vi "v6.1.vi"() -> ()   [LabVIEW 2018]
uses:
  <vilib>/DAQmx/read.llb/DAQmx Read (Analog 1D DBL NChan 1Samp).vi
  <extravilib>/ChannelInstances/Lossy Stream-c(a[.](c(dbl,dbl,dbl,dbl)),stamp,a[.](dbl),c(dbl,dbl,dbl,dbl,dbl,dbl,dbl))/Read With Abort.vi
  <extravilib>/ChannelInstances/High Speed Stream-c(a[.](c(dbl,dbl,dbl,dbl)),stamp,a[.](dbl),c(dbl,dbl,dbl,dbl,dbl,dbl,dbl))/_Read For Replicate.vi
  <extravilib>/ChannelInstances/Lossy Stream-c(a[.](c(dbl,dbl,dbl,dbl)),stamp,a[.](dbl),c(dbl,dbl,dbl,dbl,dbl,dbl,dbl))/Write With Abort.vi
  <extravilib>/ChannelInstances/Lossy Stream-c(a[.](c(dbl,dbl,dbl,dbl)),stamp,a[.](dbl),c(dbl,dbl,dbl,dbl,dbl,dbl,dbl))/EndpointRead.vi
  <extravilib>/ChannelInstances/Lossy Stream-c(a[.](c(dbl,dbl,dbl,dbl)),stamp,a[.](dbl),c(dbl,dbl,dbl,dbl,dbl,dbl,dbl))/Endpoint.vi
  <extravilib>/ChannelInstances/Lossy Stream-c(a[.](c(dbl,dbl,dbl,dbl)),stamp,a[.](dbl),c(dbl,dbl,dbl,dbl,dbl,dbl,dbl))/Instantiate.vi
  <extravilib>/ChannelInstances/Lossy Stream-c(a[.](c(dbl,dbl,dbl,dbl)),stamp,a[.](dbl),c(dbl,dbl,dbl,dbl,dbl,dbl,dbl))/)Channel.vi
  <resource>/ChannelSupport/_ChannelSupport/WaitIfNeeded.vi
  <extravilib>/ChannelInstances/High Speed Stream-c(a[.](c(dbl,dbl,dbl,dbl)),stamp,a[.](dbl),c(dbl,dbl,dbl,dbl,dbl,dbl,dbl))/Instantiate.vi
  <extravilib>/ChannelInstances/High Speed Stream-c(a[.](c(dbl,dbl,dbl,dbl)),stamp,a[.](dbl),c(dbl,dbl,dbl,dbl,dbl,dbl,dbl))/)Channel.vi
  <extravilib>/ChannelInstances/High Speed Stream-c(a[.](c(dbl,dbl,dbl,dbl)),stamp,a[.](dbl),c(dbl,dbl,dbl,dbl,dbl,dbl,dbl))/Abort Signal/Init Signal.vi
  <vilib>/Utility/file.llb/Write Delimited Spreadsheet (string).vi
  <vilib>/DAQmx/create/channels.llb/DAQmx Create Channel (AI-Temperature-Thermocouple).vi
  <vilib>/DAQmx/configure/timing.llb/DAQmx Timing (Sample Clock).vi
  <vilib>/DAQmx/miscellaneous.llb/DAQmx Fill In Error Info.vi
  <extravilib>/ChannelInstances/High Speed Stream-c(a[.](c(dbl,dbl,dbl,dbl)),stamp,a[.](dbl),c(dbl,dbl,dbl,dbl,dbl,dbl,dbl)).lvlib
  <resource>/objmgr/daqmx.rc
  <extravilib>/ChannelInstances/Lossy Stream-c(a[.](c(dbl,dbl,dbl,dbl)),stamp,a[.](dbl),c(dbl,dbl,dbl,dbl,dbl,dbl,dbl)).lvlib
panel:
  out "Driving Variables":T1
  in  "Line Controls\n(Don't Delete)":enum32{"Flowrate", "Temperatures", "Pressures"}(tab)
  in  "Line Flowrate Control":T2 {"Line 5" scale=0.0..10.0; "Line 4" scale=0.0..10.0; "Line 3" scale=0.0..10.0; "Line 2" scale=0.0..10.0; "Line 1" scale=0.0..10.0}
  in  "Temperatures Control":T2 {"Line 5" scale=0.0..10.0; "Line 4" scale=0.0..10.0; "Line 3" scale=0.0..10.0; "Line 2" scale=0.0..10.0; "Line 1" scale=0.0..10.0}
  in  "Pressure Controls":T2 {"Line 5" scale=0.0..10.0; "Line 4" scale=0.0..10.0; "Line 3" scale=0.0..10.0; "Line 2" scale=0.0..10.0; "Line 1" scale=0.0..10.0}
  in  "Rig Temperature Tab Box\n(Don't Delete)":enum32{"Rig Temps Live", "Alarm Thresholds"}(tab)
  out "Rig Temperatures":T3
  in  "Rig Alarm Thresholds":T3
  out "DAQ Current Time":timestamp format="%<%X>T"
  in  "UI Refresh Rate (Hz)":u32=1 min=1 max=500 step=1
  out "Line Pressures":T4(graph)
  out "Line Temperatures":T4(graph)
  in  "Species List":string[][](table)=[["Custom", "9999999999", ""], ["Methanol", "6.47", "19.93"], ["Butanol", "11.2", "33.075"], ["Propane", "15.67", "46.35"], ["Methane", "13.19", "50.00"], ["Hydrogen", "34.3", "119.96"], ["Ammonia", "6.0466", "22.5"], ["Pentane", "15.32", "45.36"], ["Butane", "14.98", "45.75"], ["Hexane", "15.24", "44.75"], ["Ethanol", "9", "26.70"], ["Empty (Not Used)", "0", "0"]]
  in  "Lines Tab Control\n(Don't delete)":enum32{"Live Data", "AFR Info", "Setup Lines"}(tab)
  out "Flowrate Data":T5(array[cluster])
  out "AFR Display":T6(array[cluster])
  in  "Line Setup":T7(array[cluster])
  out "Actual Sample Rate":dbl
  out "Export Timestamp":timestamp format="%<%H:%M:%S>T"
  out "UI Timestamp":timestamp format="%<%X\n%x>T"
  in  "file path (dialog if empty)":path
  out "Export Loop Status":T8(ring)
  in  "Start Recording?":bool
  in  "Stop Recording?":bool
  out "Aquisition Loop Status":T9(ring)
  in  "OK Button":bool
  in  "DAQ Properties":cluster{"Sample Rate [Hz]":dbl}={"Sample Rate [Hz]"=1.0} {"Sample Rate [Hz]" min=1.0 max=500.0 step=1.0}
  # "Loop Status"
  # "Rig Temperatures [ °C]"
  # "Rig Alarm Thresholds [ °C]"
  # "Live \n Live Line Data"
  # "Air-to-Fuel Ratios for each Line"
  # "Line Setup"
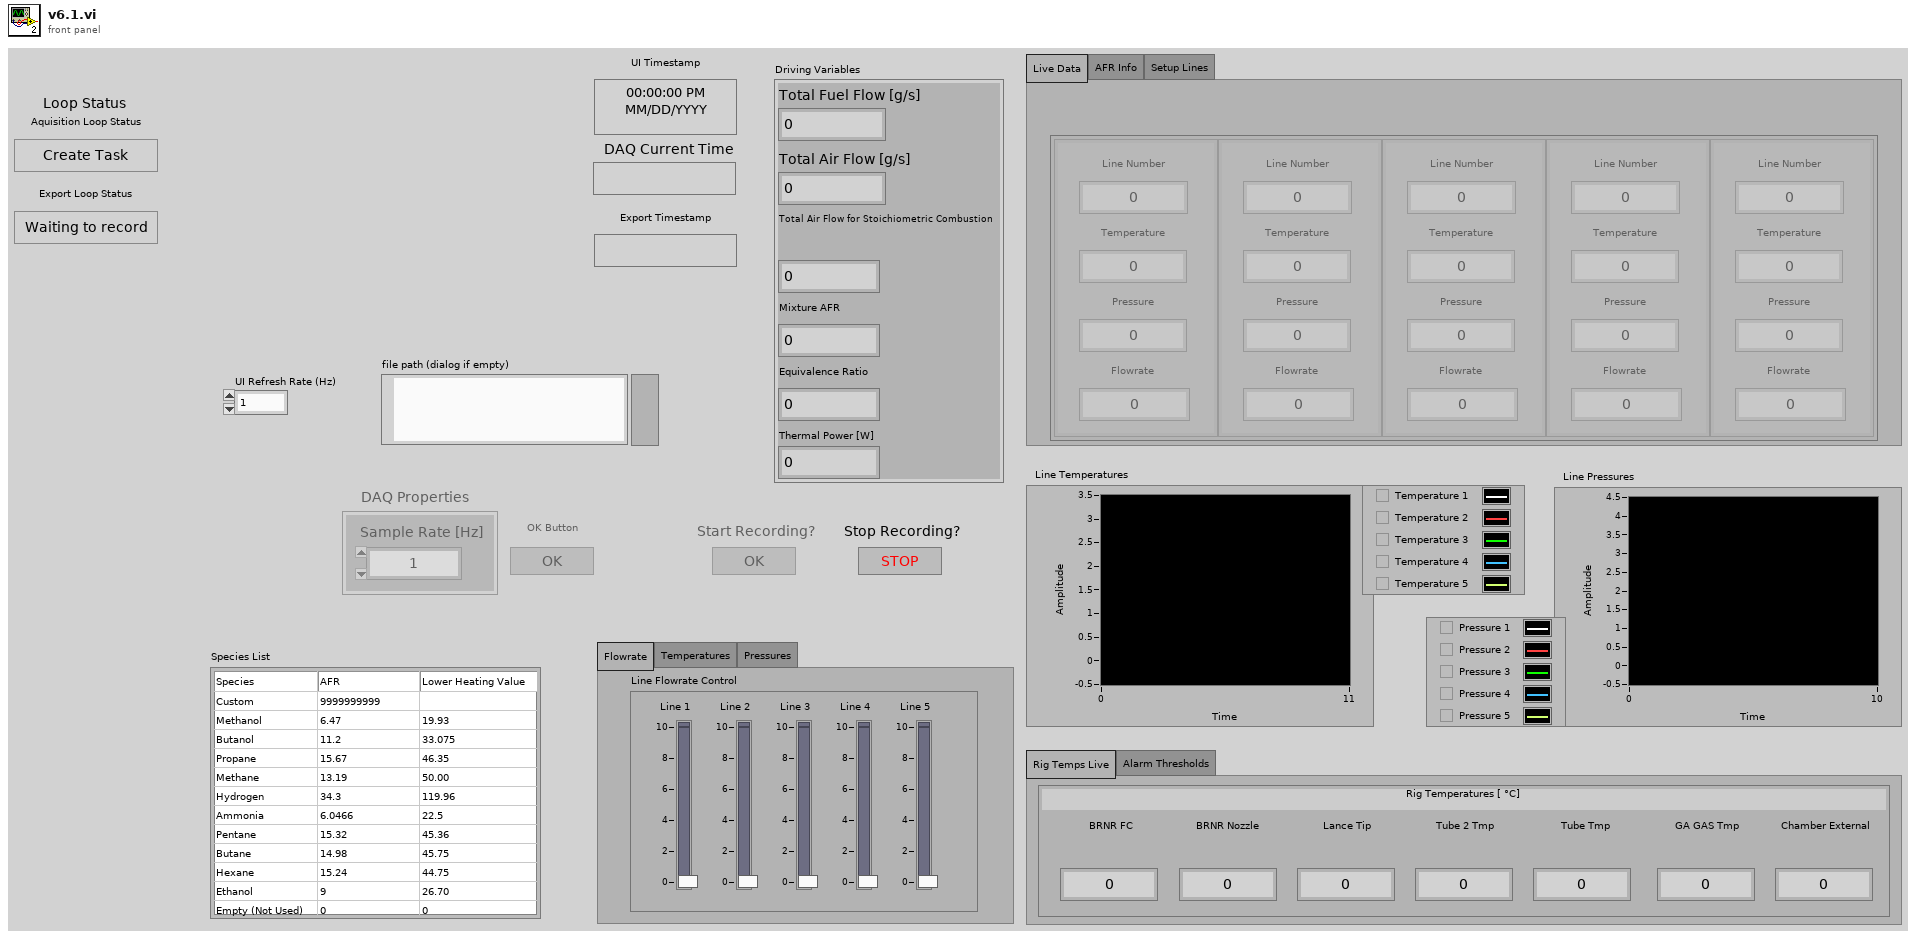
[diagram p1: front panel]
types:
  T1 = cluster{"Total Air Flow [g/s]":dbl, "Total Fuel Flow [g/s]":dbl, "Mixture AFR":dbl, "Total Air Flow for Stoichiometric Combustion":dbl, "Equivalence Ratio":dbl, "Thermal Power [W]":dbl}
  T2 = cluster{"Line 1":dbl, "Line 2":dbl, "Line 3":dbl, "Line 4":dbl, "Line 5":dbl}
  T3 = cluster{"BRNR FC":dbl, "BRNR Nozzle":dbl, "Lance Tip":dbl, "Tube 2 Tmp":dbl, "Tube Tmp":dbl, "GA GAS Tmp":dbl, "Chamber External":dbl}
  T4 = cluster{"[0]":dbl, "[1]":dbl, "[2]":dbl, "[3]":dbl, "[4]":dbl}
  T5 = cluster{"Line Number":dbl, "Temperature":dbl, "Pressure":dbl, "Flowrate":dbl}[]
  T6 = cluster{"Line Number":i32, "AFR":dbl, "Species":enum16{"Empty (Not used)", "Custom", "Air", "Methanol", "Ethanol", "Butanol", "Propane", "Methane", "Hydrogen", "Pentane", "Butane", "Hexane"}}[]
  T7 = cluster{"Custom AFR":dbl, "Species":enum16{"Empty (Not used)", "Custom", "Air", "Methanol", "Ethanol", "Butanol", "Propane", "Methane", "Hydrogen", "Pentane", "Butane", "Hexane"}, "Custom Lower Heating Value [kJ/kg]":dbl}[]
  T8 = enum16{"Waiting to record", "Creating Spreadsheet", "Recording", "Finished Recording"}
  T9 = enum16{"Create Task", "Change Settings", "Check Settings", "Read Data", "End Task"}
  T10 = enum8{"Enabled", "Disabled", "Disabled and Grayed Out"}
  T11 = cluster{"Flowrate Data":cluster{"Line Number":dbl, "Temperature":dbl, "Pressure":dbl, "Flowrate":dbl}[], "Current Time":timestamp, "DAQmx Data":dbl[], "Rig Temperatures":cluster{"BRNR FC":dbl, "BRNR Nozzle":dbl, "Lance Tip":dbl, "Tube 2 Tmp":dbl, "Tube Tmp":dbl, "GA GAS Tmp":dbl, "Chamber External Temp":dbl}}
  T12 = cluster{"BRNR FC":dbl, "BRNR Nozzle":dbl, "Lance Tip":dbl, "Tube 2 Tmp":dbl, "Tube Tmp":dbl, "GA GAS Tmp":dbl, "Chamber External Temp":dbl}
  T13 = typedef "High Speed Stream-c(a[.](c(dbl,dbl,dbl,dbl)),stamp,a[.](dbl),c(dbl,dbl,dbl,dbl,dbl,dbl,dbl)).lvlib/)Channel.ctl" = refnum<queue>
  T14 = typedef "Lossy Stream-c(a[.](c(dbl,dbl,dbl,dbl)),stamp,a[.](dbl),c(dbl,dbl,dbl,dbl,dbl,dbl,dbl)).lvlib/)Channel.ctl" = refnum<queue>
  T15 = cluster{"Line":i32, "AFR":dbl, "Species":enum16{"Empty (Not used)", "Custom", "Air", "Methanol", "Ethanol", "Butanol", "Propane", "Methane", "Hydrogen", "Pentane", "Butane", "Hexane"}}
  T16 = enum16{"Empty (Not used)", "Custom", "Air", "Methanol", "Ethanol", "Butanol", "Propane", "Methane", "Hydrogen", "Pentane", "Butane", "Hexane"}
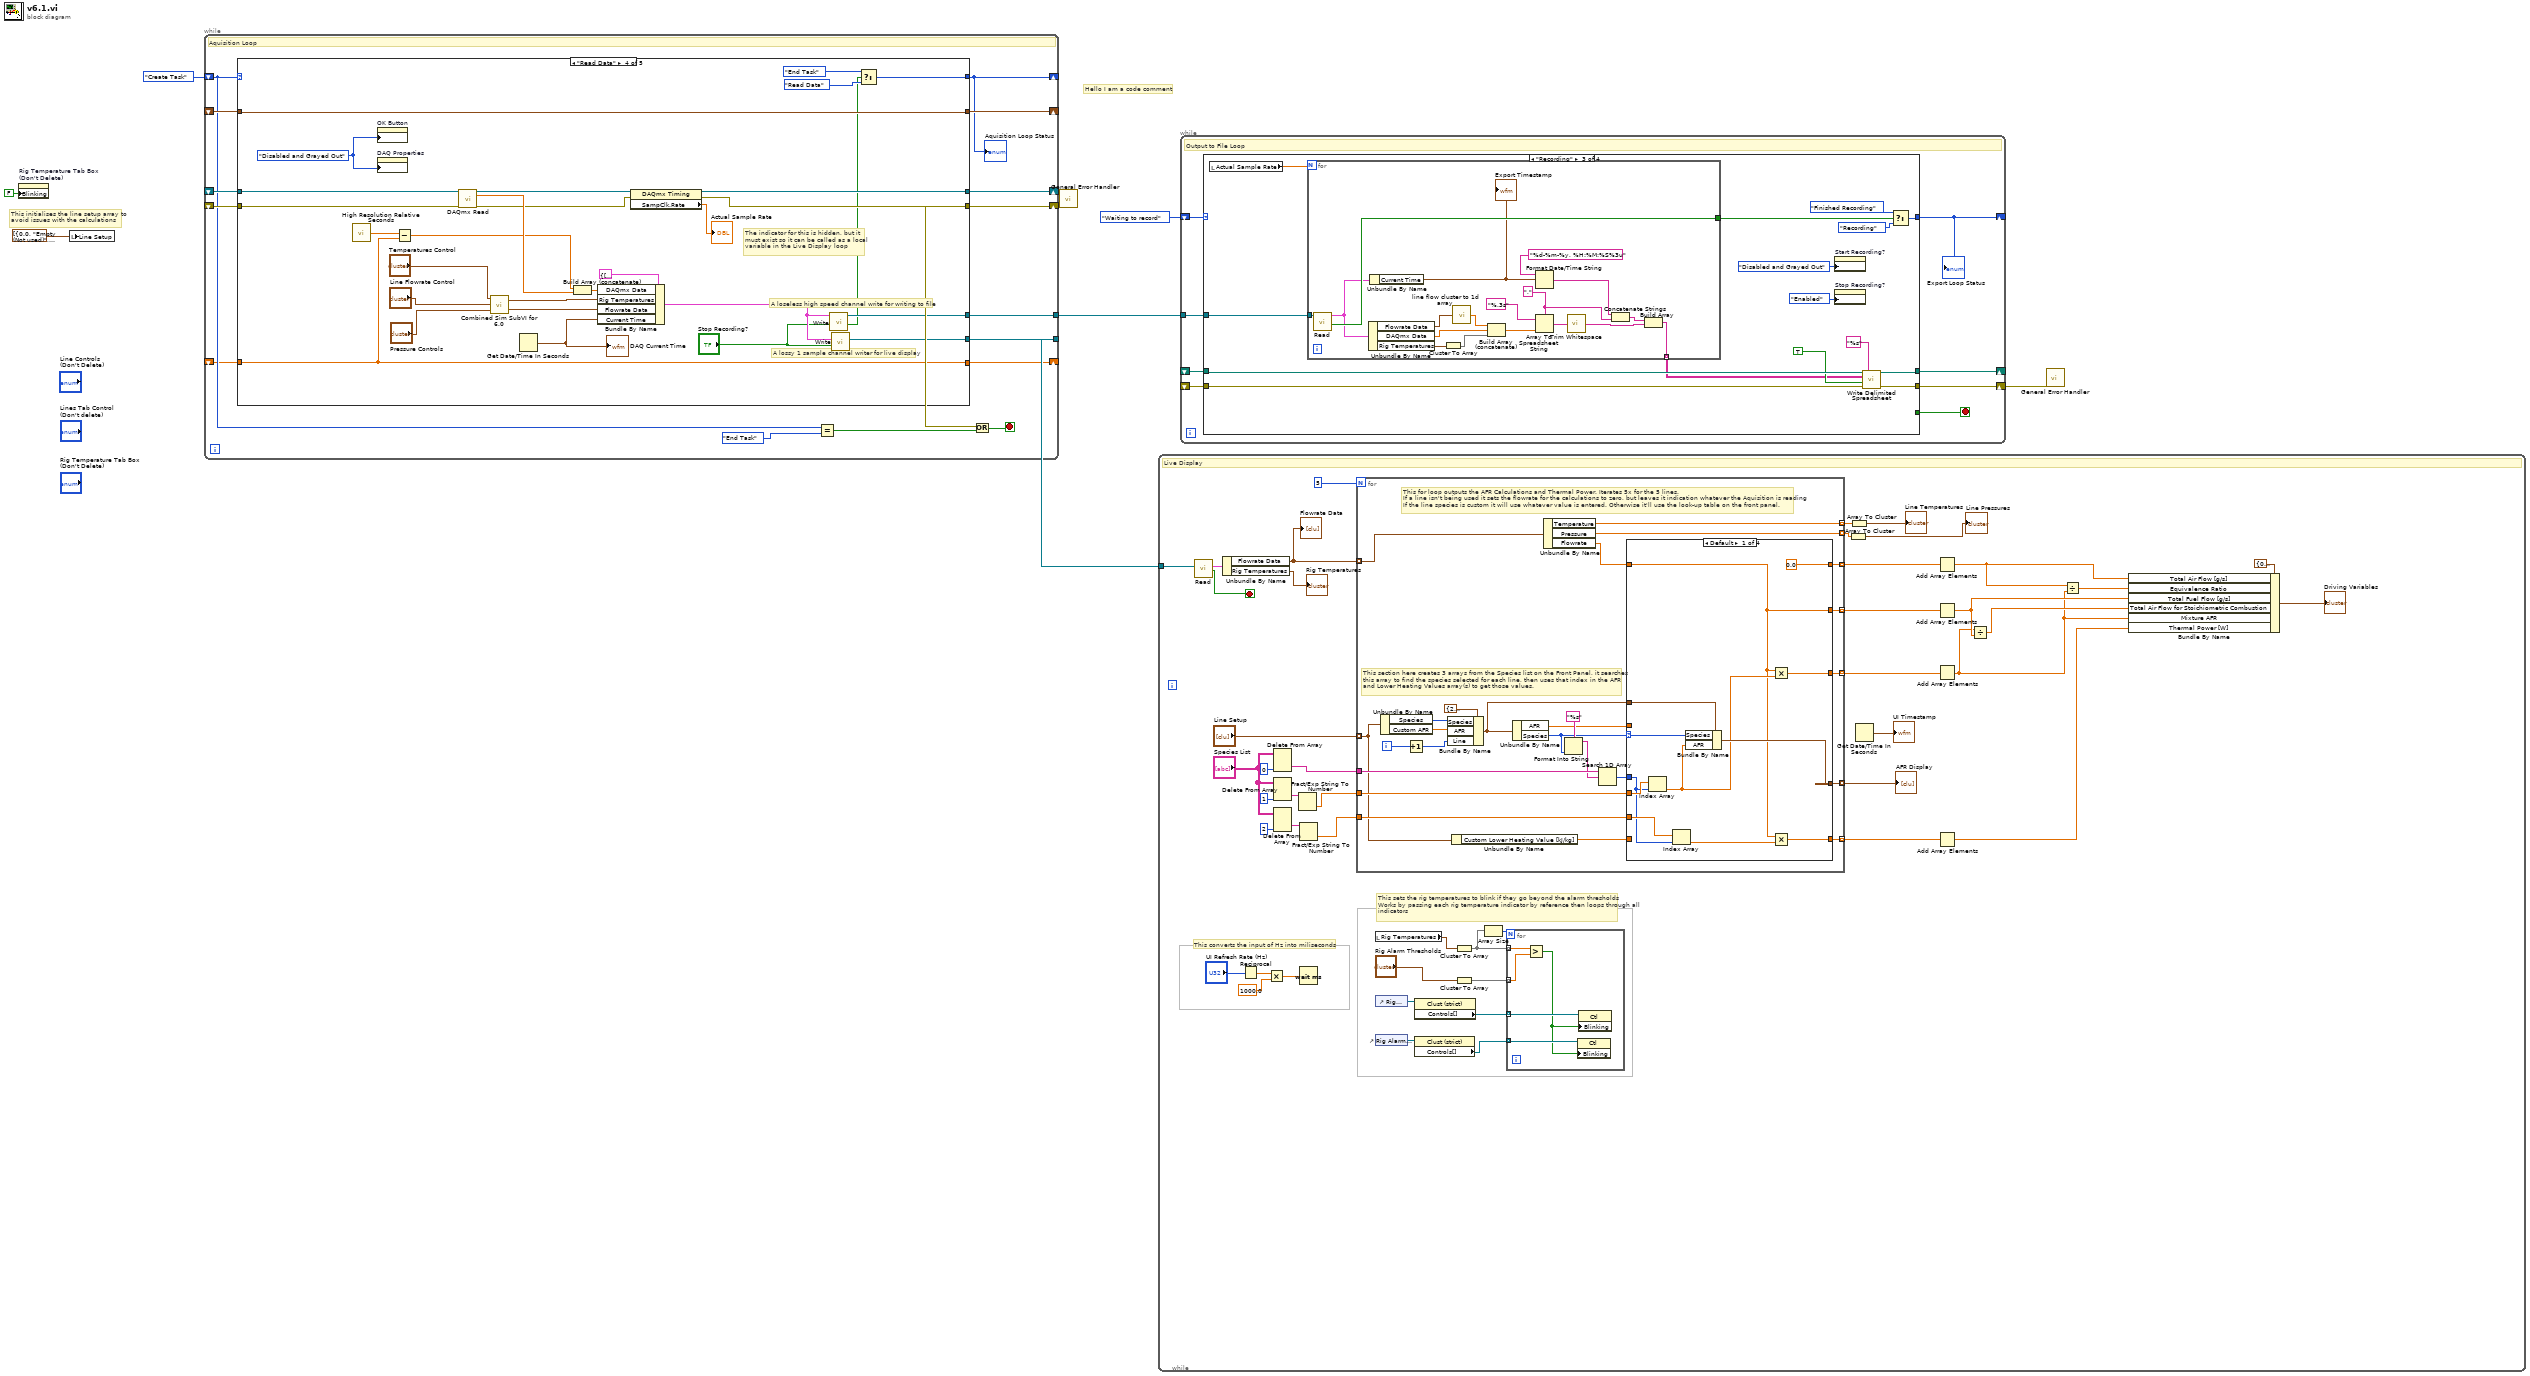
[diagram p0: block diagram]
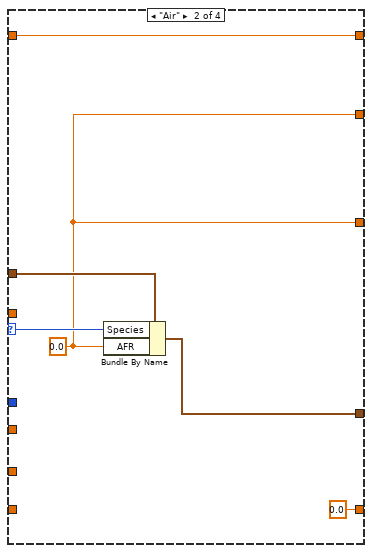
[diagram p2: hidden frame]
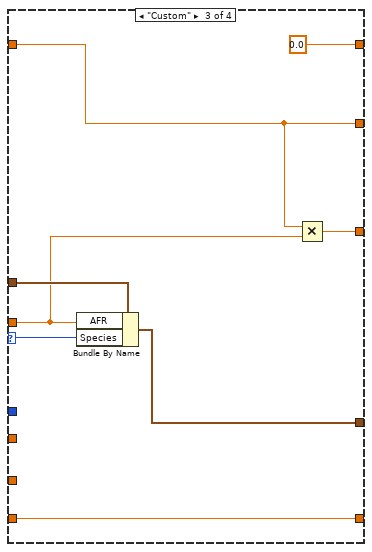
[diagram p3: hidden frame]
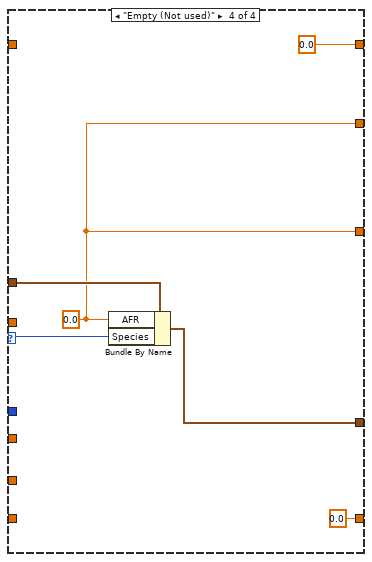
[diagram p4: hidden frame]
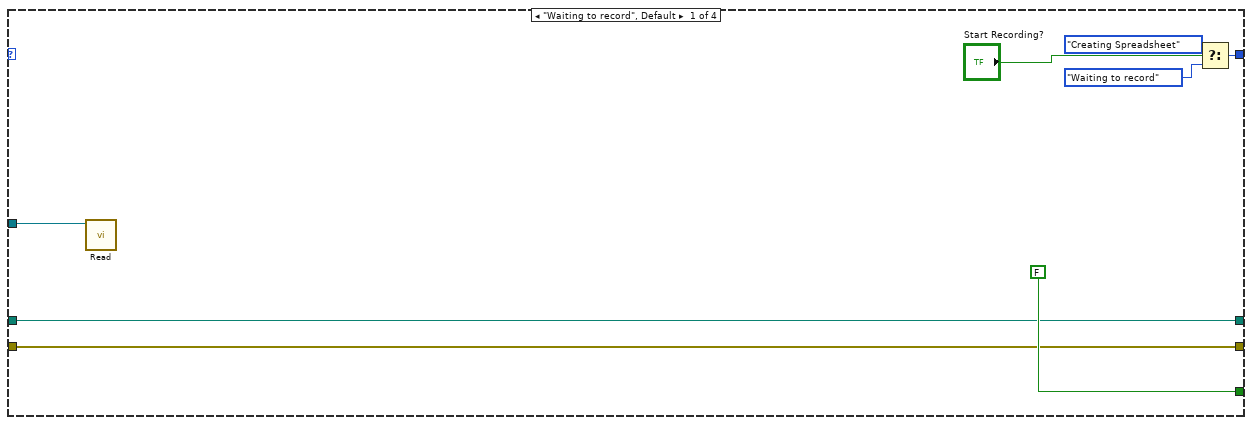
[diagram p5: hidden frame]
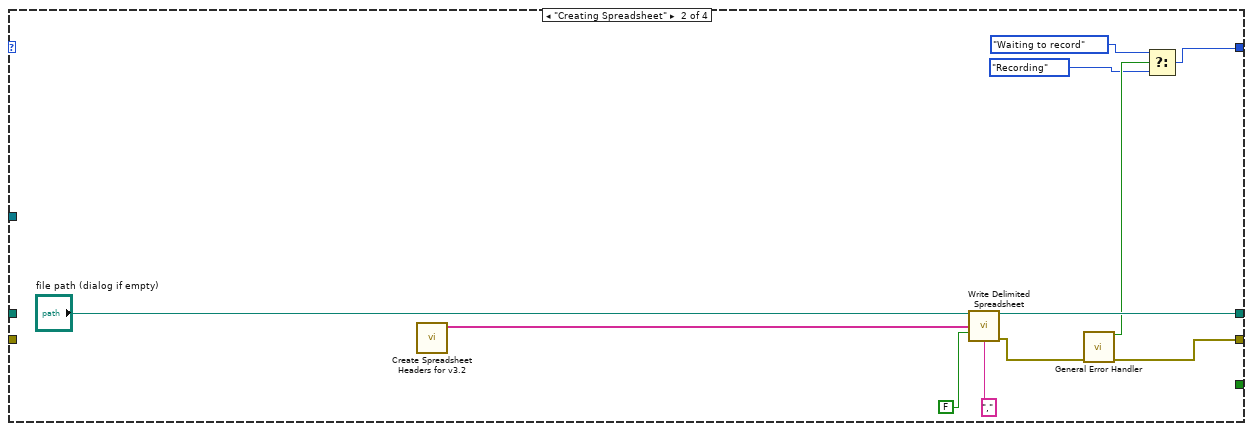
[diagram p6: hidden frame]
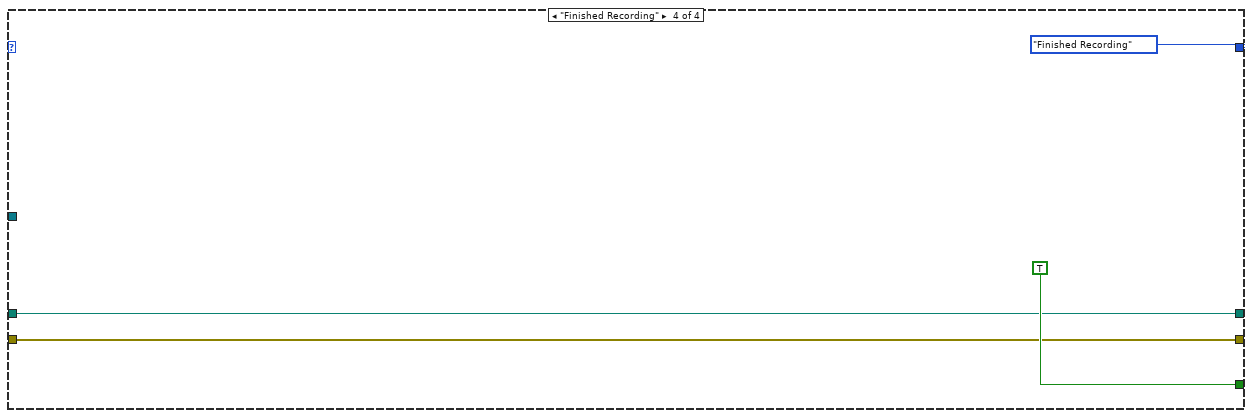
[diagram p7: hidden frame]
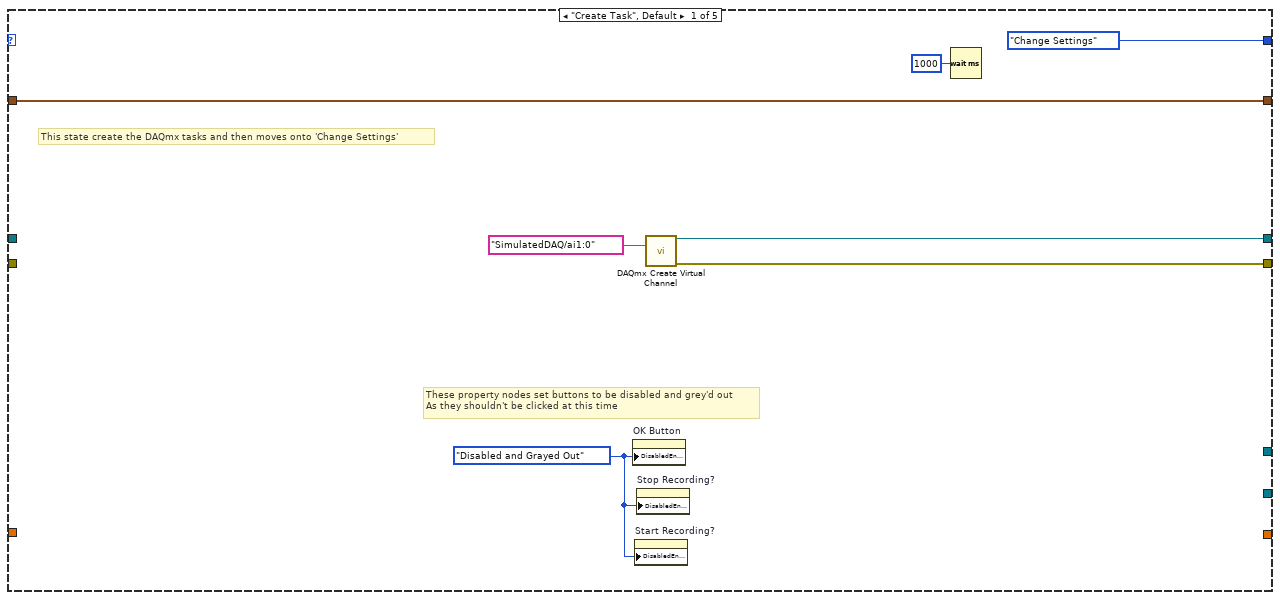
[diagram p8: hidden frame]
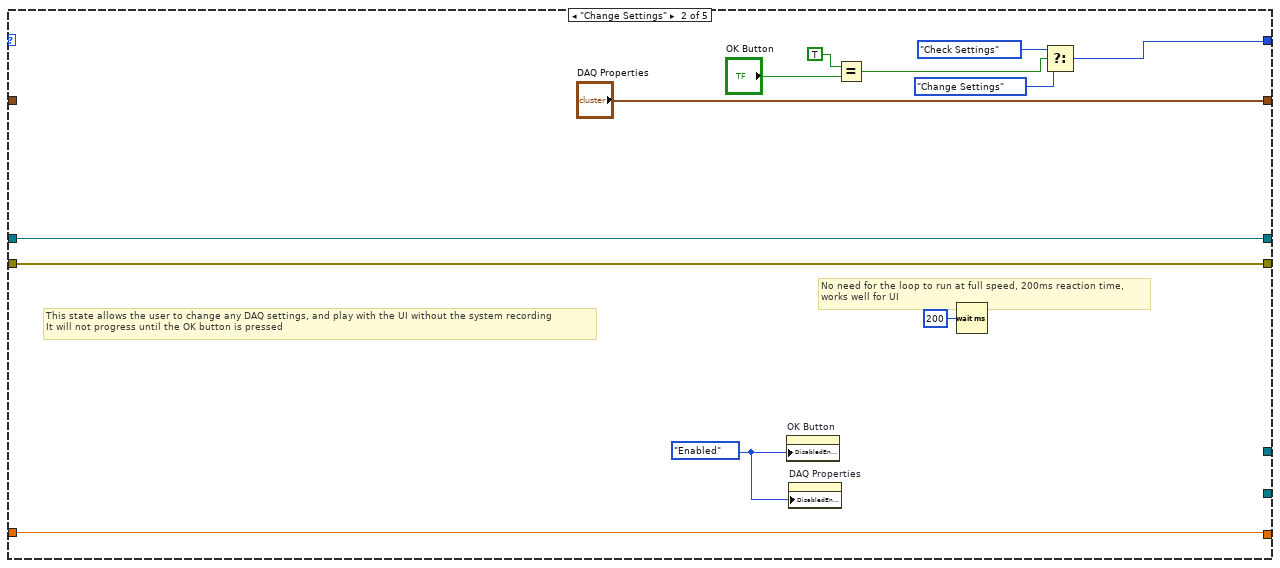
[diagram p9: hidden frame]
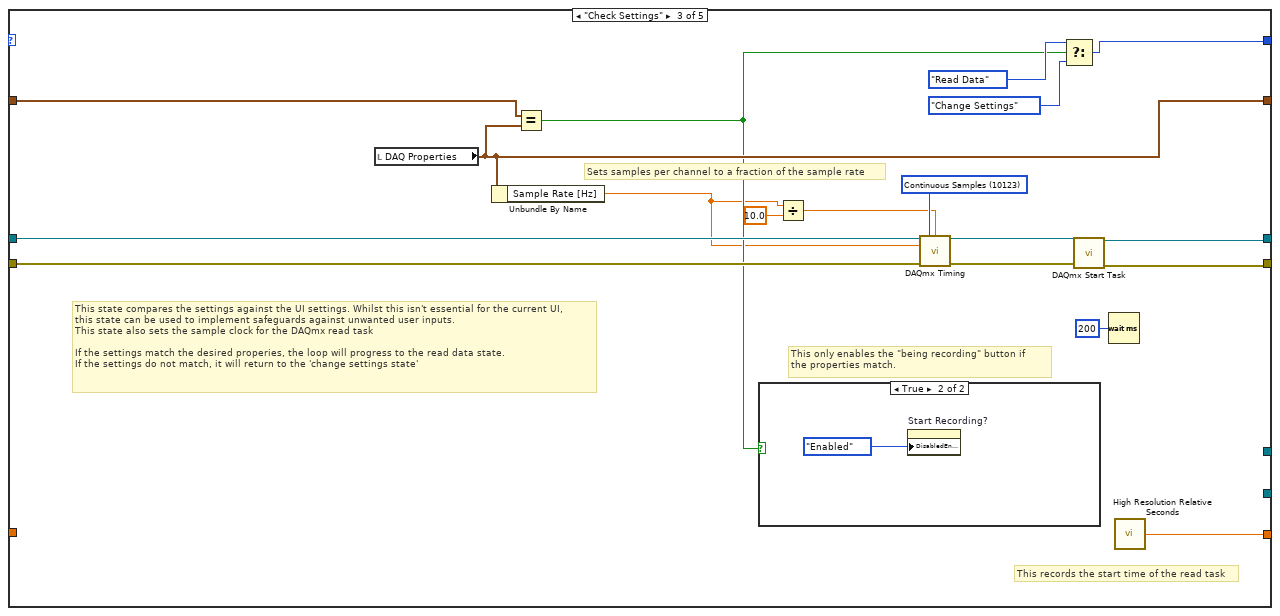
[diagram p10: hidden frame]
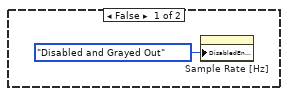
[diagram p11: hidden frame]
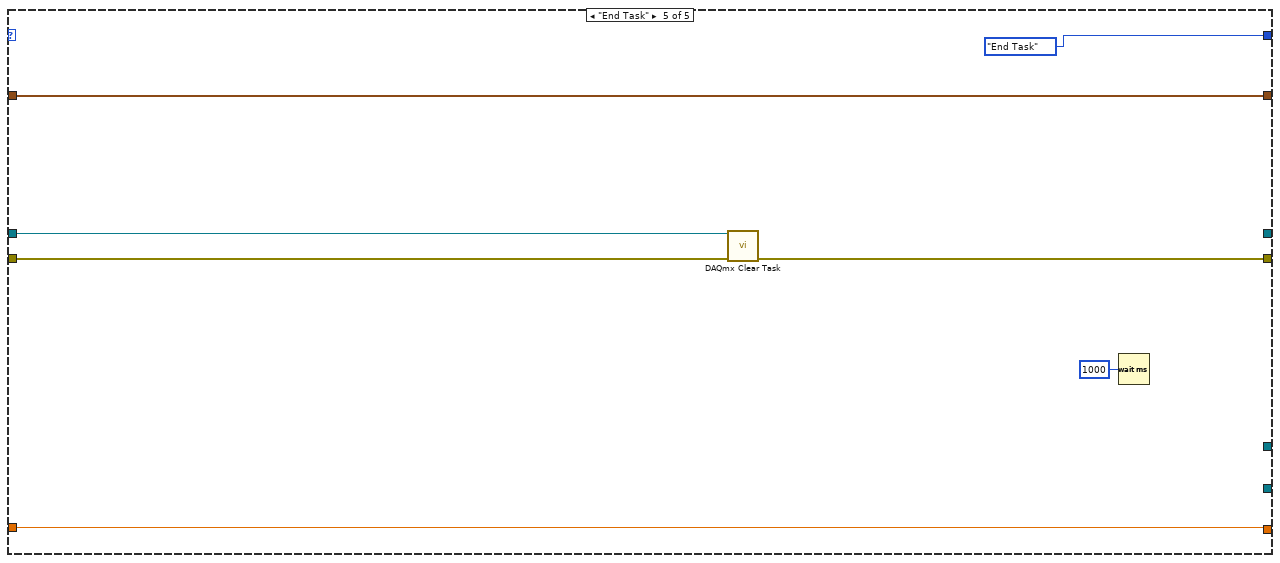
[diagram p12: hidden frame]
diagram:
  # "Hello I am a code comment"
  # "This initialises the line setup array to\navoid issues with the calculations"
  n1 = property on="Rig Temperature Tab Box\n(Don't Delete)" class="TabCtl (strict)"("Blinking"=FALSE) -> ()  [unwired: 2 in, 2 out]
  n2 = local write "Line Setup"(T7 [{"Custom AFR"=0.0, "Species"=enum."Empty (Not used)", "Custom Lower Heating Value [kJ/kg]"=0.0}, {"Custom AFR"=0.0, "Species"=enum."Empty (Not used)", "Custom Lower Heating Value [kJ/kg]"=0.0}, {"Custom AFR"=0.0, "Species"=enum."Empty (Not used)", "Custom Lower Heating Value [kJ/kg]"=0.0}, {"Custom AFR"=0.0, "Species"=enum."Empty (Not used)", "Custom Lower Heating Value [kJ/kg]"=0.0}, {"Custom AFR"=0.0, "Species"=enum."Empty (Not used)", "Custom Lower Heating Value [kJ/kg]"=0.0}] ("Line Setup")) -> ()
  n3 = while {
    shift-right: [w18] -> _
    shift-left: T9."Create Task" -> [w14]
    shift-right: [w23] -> _
    shift-left: _ -> [w21]
    shift-right: [w17] -> w4
    shift-left: _ -> [w20]
    shift-right: [w22] -> _
    shift-left: _ -> [w19]
    tunnel: [w13] -> w6
    tunnel: [w11] -> w3
    shift-right: [w9] -> _
    shift-left: _ -> [w10]
    stop <- w12 stop-if-true
    # "Aquisition Loop"
    n4 = case shown="\"Read Data\"" w14 {
      tunnel: [w30 w42 w50 w78 _] -> w23
      tunnel: [w29 w41 w49 w79 w98] -> w17
      tunnel: [T9."Change Settings" w35 w56 w87 T9."End Task"] -> w18
      tunnel: [w26 "DAQ Properties" w53 w89 w97] -> w22
      tunnel: w21 -> [_ w42 w55 w91 w95]
      tunnel: w20 -> [_ w41 w54 w90 w94]
      tunnel: w19 -> [w26 _ w60 w89 w97]
      tunnel: [_ _ _ w83 _] -> w13
      tunnel: [_ w31 w43 w74 w92] -> w9
      tunnel: w10 -> [_ w31 _ w74 w92]
      tunnel: [_ _ _ w71 _] -> w11
      frame "Create Task", Default {
        w24 = T10."Disabled and Grayed Out" ("Disabled")
        # "These property nodes set buttons to be disabled and grey'd out\nAs they shouldn't be clicked at this time"
        # "This state create the DAQmx tasks and then moves onto 'Change Settings'"
        n5 = property on="OK Button" class="Bool"("DisabledEnum"=w24) -> ()  [unwired: 2 in, 2 out]
        n6 = property on="Start Recording?" class="Bool"("DisabledEnum"=w24) -> ()  [unwired: 2 in, 2 out]
        n7 = property on="Stop Recording?" class="Bool"("DisabledEnum"=w24) -> ()  [unwired: 2 in, 2 out]
        n8 = call-poly <vilib>:"DAQmx Create Virtual Channel.vi"("physical channels"=tag "SimulatedDAQ/ai1:0") -> ("task out"=w30:refnum<k21>, "error out"=w29:errorcluster)  [unwired: 13 in]
        n9 = Wait (ms)(milliseconds to wait=u32 1000) -> ()  [unwired: 1 out]
      }
      frame "Change Settings" {
        w32 = T10."Enabled" ("Disabled")
        # "No need for the loop to run at full speed, 200ms reaction time,\nworks well for UI"
        # "This state allows the user to change any DAQ settings, and play with the UI without the system recording\nIt will not progress until the OK button is pressed"
        n10 = property on="OK Button" class="Bool"("DisabledEnum"=w32) -> ()  [unwired: 2 in, 2 out]
        n11 = property on="DAQ Properties" class="Clust (strict)"("DisabledEnum"=w32) -> ()  [unwired: 2 in, 2 out]
        n12 = Equal?(x=TRUE, y="OK Button") -> (x = y?=w37:bool)
        n13 = Wait (ms)(milliseconds to wait=u32 200) -> ()  [unwired: 1 out]
        n14 = Select(t=T9."Check Settings", s=w37, f=T9."Change Settings") -> (s? t:f=w35:T9)
      }
      frame "Check Settings" {
        w48 = 10123 items=["Finite Samples"=10178, "Continuous Samples"=10123, "Hardware Timed Single Point"=12522] ("sample mode")
        # "This records the start time of the read task"
        # "This only enables the \"being recording\" button if \nthe properties match."
        # "Sets samples per channel to a fraction of the sample rate"
        # "This state compares the settings against the UI settings. Whilst this isn't essential for the current UI, \nthis state can be used to implement safeguards against unwanted user inputs.\nThis state also sets the sample clock for the DAQmx read task\n\nIf the settings match the desired properies, the loop will progress to the read data state.\nIf the settings do not match, it will return to the 'change settings state'"
        n15 = local read "DAQ Properties"() -> (w53:cluster{"Sample Rate [Hz]":dbl})
        n16 = Unbundle By Name(w53) -> ("Sample Rate [Hz]"=w45:dbl)
        n17 = Equal?(x=w60, y=w53) -> (x = y?=w47:bool)
        n18 = case shown="True" w47 {
          frame False {
            n19 = property on="Sample Rate [Hz]" class="DigNum (strict)"("DisabledEnum"=T10."Disabled and Grayed Out" ("Disabled")) -> ()  [unwired: 2 in, 2 out]
          }
          frame True {
            n20 = property on="Start Recording?" class="Bool"("DisabledEnum"=T10."Enabled" ("Disabled")) -> ()  [unwired: 2 in, 2 out]
          }
        }
        n21 = Divide(x=w45, y=10.0) -> (x/y=w44:dbl)
        n22 = call-poly <vilib>:"DAQmx Timing.vi"("task/channels in"=w55, "sample mode"=w48, "samples per channel"=w44, "rate"=w45, "error in"=w54) -> ("task out"=w52:refnum<k21>, "error out"=w51:errorcluster)  [unwired: 9 in]
        n23 = Select(t=T9."Read Data", s=w47, f=T9."Change Settings") -> (s? t:f=w56:T9)
        n24 = call <vilib>:"DAQmx Start Task.vi"("task/channels in"=w52, "error in"=w51) -> ("task out"=w50:refnum<k21>, "error out"=w49:errorcluster)  [unwired: 12 in]
        n25 = Wait (ms)(milliseconds to wait=u32 200) -> ()  [unwired: 1 out]
        n26 = call <vilib>:"High Resolution Relative Seconds.vi"() -> ("relative seconds"=w43:dbl)
      }
      frame "Read Data" {
        w82 = T10."Disabled and Grayed Out" ("Disabled")
        # "A lossy 1 sample channel writer for live display"
        # "A loseless high speed channel write for writing to file"
        # "The indicator for this is hidden, but it\nmust exist so it can be called as a local \nvariable in the Live Display loop"
        n27 = call <vilib>:"High Resolution Relative Seconds.vi"() -> ("relative seconds"=w76:dbl)
        n28 = property on="OK Button" class="Bool"("DisabledEnum"=w82) -> ()  [unwired: 2 in, 2 out]
        n29 = property on="DAQ Properties" class="Clust (strict)"("DisabledEnum"=w82) -> ()  [unwired: 2 in, 2 out]
        n30 = Subtract(x=w76, y=w74) -> (x-y=w75:dbl)
        n31 = call-poly <vilib>:"DAQmx Read.vi"("task/channels in"=w91, "error in"=w90) -> ("task out"=w80:refnum<k21>, "data"=w85:dbl[], "error out"=w77:errorcluster)  [unwired: 11 in]
        n32 = call "Combined Sim SubVI for 6.0.vi"("Pressure Controls"="Pressure Controls", "Line Flowrate Control"="Line Flowrate Control", "Temperatures Control"="Temperatures Control") -> ("Array"=w66:T5, "Cluster"=w67:T12)
        n33 = Get Date/Time In Seconds() -> (seconds since 1Jan1904=w68:timestamp)
        "DAQ Current Time" <- w68
        n34 = Build Array (concatenate)(w75, w85) -> (w69:dbl[])
        n35 = Bundle By Name(cluster=T11 {"Flowrate Data"=[{"Line Number"=1.0, "Temperature"=17.480721541683437, "Pressure"=24.0, "Flowrate"=0.0}, {"Line Number"=2.0, "Temperature"=21.850901927104296, "Pressure"=30.0, "Flowrate"=0.0}, {"Line Number"=3.0, "Temperature"=26.221082312525155, "Pressure"=36.0, "Flowrate"=0.0}, {"Line Number"=4.0, "Temperature"=30.591262697946018, "Pressure"=42.00000000000001, "Flowrate"=0.0}, {"Line Number"=5.0, "Temperature"=34.96144308336687, "Pressure"=48.0, "Flowrate"=0.0}], "Current Time"=timestamp(0 s since 1904-01-01), "DAQmx Data"=[], "Rig Temperatures"={"BRNR FC"=0.0, "BRNR Nozzle"=0.0, "Lance Tip"=0.0, "Tube 2 Tmp"=0.0, "Tube Tmp"=0.0, "GA GAS Tmp"=0.0, "Chamber External Temp"=0.0}}, "DAQmx Data"=w69, "Rig Temperatures"=w67, "Flowrate Data"=w66, "Current Time"=w68) -> (w81:T11)
        n36 = property class="DAQmx Timing"(reference=w80, error in=w77) -> (reference out=w78:refnum<k21>, error out=w79:errorcluster, "SampClk.Rate"=→"Actual Sample Rate":dbl)
        n37 = call <extravilib>:"Write.vi"("last element? (F)"="Stop Recording?", "element"=w81) -> ("done?"=w70:bool, "channel"=w83:T13)  [unwired: 7 in, 1 out]
        n38 = call <extravilib>:"Write.vi"("last element? (F)"="Stop Recording?", "element"=w81) -> ("channel"=w71:T14)  [unwired: 7 in, 2 out]
        n39 = Select(t=T9."End Task", s=w70, f=T9."Read Data") -> (s? t:f=w87:T9)
      }
      frame "End Task" {
        n40 = call <vilib>:"DAQmx Clear Task.vi"("task in"=w95, "error in"=w94) -> ("error out"=w98:errorcluster)  [unwired: 13 in]
        n41 = Wait (ms)(milliseconds to wait=u32 1000) -> ()  [unwired: 1 out]
      }
    }
    "Aquisition Loop Status" <- w18
    n42 = Equal?(x=w14, y=T9."End Task") -> (x = y?=w15:bool)
    n43 = Or(x=w17, y=w15) -> (x .or. y?=w12:bool)
  }
  n44 = call <vilib>:"General Error Handler.vi"("error in (no error)"=w4) -> ()  [unwired: 10 in, 5 out]
  n45 = while {
    tunnel: w3 -> [w144]
    stop <- w141 stop-if-true
    # "This converts the input of Hz into miliseconds"
    # "This sets the rig temperatures to blink if they go beyond the alarm thresholds\nWorks by passing each rig temperature indicator by reference then loops through all indicators"
    # "Live Display"
    n46 = call <extravilib>:"Read.vi"("channel"=w144) -> ("last element?"=w141:bool, "element"=w143:T11)  [unwired: 5 in, 4 out]
    n47 = Unbundle By Name(w143) -> ("Flowrate Data"=w123:T5, "Rig Temperatures"=→"Rig Temperatures":T12)
    "Flowrate Data" <- w123
    n48 = Reciprocal(x="UI Refresh Rate (Hz)") -> (1/x=w109:dbl)
    n49 = Multiply(x=w109, y=1000.0) -> (x*y=w139:dbl)
    n50 = Delete From Array(array="Species List", index (col)=0) -> (deleted portion=w134:string[])  [unwired: 2 in, 1 out]
    n51 = Delete From Array(array="Species List", index (col)=1 ("disabled index (col)")) -> (deleted portion=w135:string[])  [unwired: 2 in, 1 out]
    n52 = Delete From Array(array="Species List", index (col)=2 ("disabled index (col)")) -> (deleted portion=w111:string[])  [unwired: 2 in, 1 out]
    n53 = Fract/Exp String To Number(string=w135) -> (number=w136:dbl[])  [unwired: 3 in, 1 out]
    n54 = Fract/Exp String To Number(string=w111) -> (number=w110:dbl[])  [unwired: 3 in, 1 out]
    n55 = Wait (ms)(milliseconds to wait=w139) -> ()  [unwired: 1 out]
    n56 = for {
      N: 5 -> [_]
      tunnel: w134 -> [w174]
      tunnel: w136 -> [w171]
      tunnel: "Line Setup" -> [w152] mode=indexing
      tunnel: [w162] -> w138 mode=indexing
      tunnel: w123 -> [w156] mode=indexing
      tunnel: [w161] -> w130 mode=indexing
      tunnel: [w160] -> w128 mode=indexing
      tunnel: [w158] -> w126 mode=indexing
      tunnel: [w157] -> w125 mode=indexing
      tunnel: [w155] -> w124 mode=indexing
      tunnel: w110 -> [w154]
      tunnel: [w153] -> w99 mode=indexing
      i -> [w164]
      # "This section here creates 3 arrays from the Species list on the Front Panel, it searches \nthis array to find the species selected for each line, then uses that index in the AFR \nand Lower Heating Values array(s) to get those values."
      # "This for loop outputs the AFR Calculations and Thermal Power. Iterates 5x for the 5 lines.\nIf a line isn't being used it sets the flowrate for the calculations to zero, but leaves it indication whatever the Aquisition is reading\nIf the line species is custom it will use whatever value is entered. Otherwise it'll use the look-up table on the front panel."
      n57 = Unbundle By Name(w152) -> ("Species"=w168:T16, "Custom AFR"=w167:dbl)
      n58 = Increment(x=w164) -> (x+1=w165:i32)
      n59 = Bundle By Name(cluster=T15 {"Line"=2, "AFR"=1.0, "Species"=enum."Butane"} ("AFR Inputs"), "Species"=w168, "AFR"=w167, "Line"=w165) -> (w163:T15)
      n60 = Unbundle By Name(w152) -> ("Custom Lower Heating Value [kJ/kg]"=w151:dbl)
      n61 = Unbundle By Name(w163) -> ("AFR"=w172:dbl, "Species"=w169:T16)
      n62 = Unbundle By Name(w156) -> ("Temperature"=w161:dbl, "Pressure"=w160:dbl, "Flowrate"=w159:dbl)
      n63 = Format Into String(format string="%s", w169) -> (resulting string=w173:string)  [unwired: 2 in, 1 out]
      n64 = Search 1D Array(1D array=w174, element=w173) -> (index of element=w170:i32)  [unwired: 1 in]
      n65 = case shown="Default" w169 {
        selector: w169 -> [w186 w193 w199 w205]
        tunnel: w172 -> [_ _ w197 _]
        tunnel: w171 -> [w187 _ _ _]
        tunnel: w170 -> [w179 _ _ _]
        tunnel: [w184 w192 w201 w207] -> w162
        tunnel: w163 -> [w185 w191 w200 w206]
        tunnel: w159 -> [w178 w190 w195 _]
        tunnel: [w182 w189 w196 w204] -> w158
        tunnel: [w178 w189 w195 w204] -> w157
        tunnel: [0.0 ("Flowrate") w190 0.0 ("Flowrate") 0.0 ("Flowrate")] -> w155
        tunnel: w154 -> [w180 _ _ _]
        tunnel: [w176 0.0 w194 0.0] -> w153
        tunnel: w151 -> [_ _ w194 _]
        frame Default {
          n66 = Index Array(array=w187, index=w179) -> (element=w183:dbl)
          n67 = Index Array(array=w180, index=w179) -> (element=w177:dbl)
          n68 = Bundle By Name(cluster=w185, "Species"=w186, "AFR"=w183) -> (w184:T15)
          n69 = Multiply(x=w178, y=w183) -> (x*y=w182:dbl)
          n70 = Multiply(x=w178, y=w177) -> (x*y=w176:dbl)
        }
        frame "Air" {
          w189 = 0.0 ("AFR")
          n71 = Bundle By Name(cluster=w191, "Species"=w193, "AFR"=w189) -> (w192:T15)
        }
        frame "Custom" {
          n72 = Bundle By Name(cluster=w200, "AFR"=w197, "Species"=w199) -> (w201:T15)
          n73 = Multiply(x=w195, y=w197) -> (x*y=w196:dbl)
        }
        frame "Empty (Not used)" {
          w204 = 0.0 ("AFR")
          n74 = Bundle By Name(cluster=w206, "AFR"=w204, "Species"=w205) -> (w207:T15)
        }
      }
    }
    "AFR Display" <- w138
    n75 = local read "Rig Temperatures"() -> (w121:T3)
    n76 = control-ref of="Rig Temperatures"() -> (w117:refnum<vi>)
    n77 = control-ref of="Rig Alarm Thresholds"() -> (w115:refnum<vi>)
    n78 = property class="Clust (strict)"(reference=w115) -> ("Controls[]"=w114:refnum<vi>[])  [unwired: 1 in, 2 out]
    n79 = property class="Clust (strict)"(reference=w117) -> ("Controls[]"=w116:refnum<vi>[])  [unwired: 1 in, 2 out]
    n80 = Cluster To Array(cluster=w121) -> (array=w118:dbl[])
    n81 = Cluster To Array(cluster="Rig Alarm Thresholds") -> (array=w120:dbl[])
    n82 = Array Size(array=w118) -> (size(s)=w119:i32)
    n83 = for {
      N: w119 -> [_]
      tunnel: w120 -> [w149] mode=indexing
      tunnel: w118 -> [w150] mode=indexing
      tunnel: w116 -> [w147] mode=indexing
      tunnel: w114 -> [w148] mode=indexing
      n84 = Greater?(x=w150, y=w149) -> (0:w146:bool)
      n85 = property on="Property Node" class="Ctl"(reference=w148, "Blinking"=w146) -> ()  [unwired: 1 in, 2 out]
      n86 = property on="Property Node" class="Ctl"(reference=w147, "Blinking"=w146) -> ()  [unwired: 1 in, 2 out]
    }
    n87 = Array To Cluster(array=w128) -> (cluster=→"Line Pressures":T4)
    n88 = Array To Cluster(array=w130) -> (cluster=→"Line Temperatures":T4)
    n89 = Get Date/Time In Seconds() -> (seconds since 1Jan1904=→"UI Timestamp":timestamp)
    n90 = Add Array Elements(numeric array=w124) -> (sum=w105:dbl)
    n91 = Add Array Elements(numeric array=w125) -> (sum=w103:dbl)
    n92 = Add Array Elements(numeric array=w126) -> (sum=w101:dbl)
    n93 = Add Array Elements(numeric array=w99) -> (sum=w100:dbl)
    n94 = Divide(x=w101, y=w103) -> (x/y=w102:dbl)
    n95 = Divide(x=w105, y=w101) -> (x/y=w104:dbl)
    n96 = Bundle By Name(cluster=T1 {"Total Air Flow [g/s]"=0.0, "Total Fuel Flow [g/s]"=0.0, "Mixture AFR"=0.0, "Total Air Flow for Stoichiometric Combustion"=0.0, "Equivalence Ratio"=0.0, "Thermal Power [W]"=0.0} ("Driving Variables 2"), "Total Air Flow [g/s]"=w105, "Equivalence Ratio"=w104, "Total Fuel Flow [g/s]"=w103, "Total Air Flow for Stoichiometric Combustion"=w102, "Mixture AFR"=w101, "Thermal Power [W]"=w100) -> (→"Driving Variables":T1)
  }
  n97 = while {
    shift-right: [w215] -> _
    shift-left: T8."Waiting to record" -> [w214]
    tunnel: w6 -> [w212]
    shift-right: [w210] -> _
    shift-left: _ -> [w211]
    shift-right: [w209] -> w5
    shift-left: _ -> [w208]
    stop <- w213 stop-if-true
    # "Output to File Loop"
    n98 = case shown="\"Recording\"" w214 {
      tunnel: [w220 w226 w248 T8."Finished Recording"] -> w215
      tunnel: [FALSE _ _ TRUE] -> w213
      tunnel: w212 -> [w216 _ w245 _]
      tunnel: w211 -> [w218 _ w242 w269]
      tunnel: [w218 w234 w243 w269] -> w210
      tunnel: [w217 w228 w238 w268] -> w209
      tunnel: w208 -> [w217 _ w241 w268]
      frame "Waiting to record", Default {
        n99 = call <extravilib>:"Read.vi"("channel"=w216) -> ()  [unwired: 6 in, 5 out]
        n100 = Select(t=T8."Creating Spreadsheet", s="Start Recording?", f=T8."Waiting to record") -> (s? t:f=w220:T8)
      }
      frame "Creating Spreadsheet" {
        n101 = call "Create Spreadsheet Headers for v3.2.vi"() -> ("Array"=w233:string[])  [unwired: 11 in]
        n102 = call-poly <vilib>:"Write Delimited Spreadsheet.vi"("file path (dialog if empty)"="file path (dialog if empty)", "1D data"=w233, "append to file? (new file:F)"=FALSE, "delimiter (\\t)"="," ("delimiter (\\t)")) -> ("new file path (Not A Path if cancelled)"=w234:path, "error out"=w229:errorcluster)  [unwired: 10 in]
        n103 = call <vilib>:"General Error Handler.vi"("error in (no error)"=w229) -> ("error?"=w227:bool, "error out"=w228:errorcluster)  [unwired: 10 in, 3 out]
        n104 = Select(t=T8."Waiting to record", s=w227, f=T8."Recording") -> (s? t:f=w226:T8)
      }
      frame "Recording" {
        n105 = local read "Actual Sample Rate"() -> (w235:dbl)
        n106 = for {
          N: w235 -> [_]
          tunnel: w245 -> [w266]
          tunnel: [w265] -> w244
          tunnel: [w250] -> w236 mode=indexing
          w255 = "," ("delimiter (Tab)")
          n107 = call <extravilib>:"Read.vi"("channel"=w266) -> ("done?"=w265:bool, "element"=w263:T11)  [unwired: 6 in, 3 out]
          n108 = Unbundle By Name(w263) -> ("Flowrate Data"=w264:T5, "DAQmx Data"=w261:dbl[], "Rig Temperatures"=w267:T12)
          n109 = Unbundle By Name(w263) -> ("Current Time"=w256:timestamp)
          "Export Timestamp" <- w256
          n110 = Cluster To Array(cluster=w267) -> (array=w262:dbl[])
          n111 = call "line flow cluster to 1d array.vi"("Flowrate Data"=w264) -> ("Array"=w260:dbl[])
          n112 = Build Array (concatenate)(w260, w261, w262) -> (w253:dbl[])
          n113 = Format Date/Time String(time format string (%c)="%d-%m-%y, %H:%M:%S%3u", seconds (now)=w256) -> (date/time string=w254:string)  [unwired: 1 in]
          n114 = Array To Spreadsheet String(delimiter (Tab)=w255, array=w253, 3:"%.3s" ("format string")) -> (spreadsheet string=w259:string)
          n115 = call <vilib>:"Trim Whitespace.vi"("string"=w259) -> ("trimmed string"=w251:string)  [unwired: 1 in]
          n116 = Concatenate Strings(w254, w255) -> (w252:string)
          n117 = Build Array(w252, w251) -> (w250:string[])
        }
        n118 = property on="Start Recording?" class="Bool"("DisabledEnum"=T10."Disabled and Grayed Out" ("Disabled")) -> ()  [unwired: 2 in, 2 out]
        n119 = property on="Stop Recording?" class="Bool"("DisabledEnum"=T10."Enabled" ("Disabled")) -> ()  [unwired: 2 in, 2 out]
        n120 = call-poly <vilib>:"Write Delimited Spreadsheet.vi"("file path (dialog if empty)"=w242, "format (%s)"="%s", "2D data"=w236, "append to file? (new file:F)"=TRUE, "error in (no error)"=w241) -> ("new file path (Not A Path if cancelled)"=w243:path, "error out"=w238:errorcluster)  [unwired: 9 in]
        n121 = Select(t=T8."Finished Recording", s=w244, f=T8."Recording") -> (s? t:f=w248:T8)
      }
      frame "Finished Recording" {
      }
    }
    "Export Loop Status" <- w215
  }
  n122 = call <vilib>:"General Error Handler.vi"("error in (no error)"=w5) -> ()  [unwired: 10 in, 5 out]
